vi "Number to West string.vi"(1 "Max decimal places desired":i32 min=0 max=3, 2 "Value":dbl min=-9999.0 max=9999.0 format="%.3f") -> (0 "West formatted value":string)   [LabVIEW 2010]
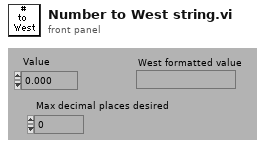
[diagram p1: front panel]
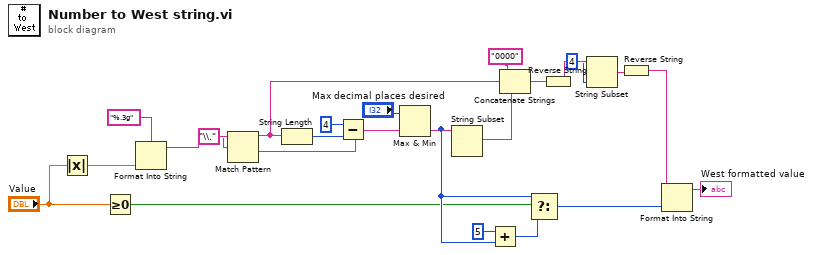
[diagram p0: block diagram]
diagram:
  n1 = Absolute Value(x="Value") -> (abs(x)=w22:dbl)
  n2 = Greater Or Equal To 0?(x="Value") -> (x >= 0?=w11:bool)
  n3 = Format Into String(format string="%.3g", w22) -> (resulting string=w24:string)  [unwired: 2 in, 1 out]
  n4 = Match Pattern(string=w24, regular expression="\\.") -> (before substring=w13:string, after substring=w19:string)  [unwired: 1 in, 2 out]
  n5 = String Length(string=w13) -> (length=w17:i32)
  n6 = Subtract(x=4, y=w17) -> (x-y=w15:i32)
  n7 = Max & Min(x="Max decimal places desired", y=w15) -> (min(x,y)=w12:i32)  [unwired: 1 out]
  n8 = String Subset(string=w19, length (rest)=w12) -> (substring=w18:string)  [unwired: 1 in]
  n9 = Add(x=5, y=w12) -> (x+y=w9:i32)
  n10 = Concatenate Strings("0000", w13, w18) -> (w6:string)
  n11 = Select(t=w12, s=w11, f=w9) -> (s? t:f=w1:i32)
  n12 = Reverse String(1:w6) -> (0:w5:string)
  n13 = String Subset(string=w5, length (rest)=4 ("length")) -> (substring=w3:string)  [unwired: 1 in]
  n14 = Reverse String(1:w3) -> (0:w2:string)
  n15 = Format Into String(initial string=w2, w1) -> (resulting string=→"West formatted value":string)  [unwired: 2 in, 1 out]
